vi "ABR3-Analyze.vi"(0 "Neural (uV)":dbl[](array[numeric]), 2 "Runtime":T1={"Ceiling"=0.0, "Threshold"=0.0, "Crossed?"=FALSE, "Step"=0, "Stop"=0, "Avgs"=0, "Level"=0.0, "AI Npts"=0, "Doubled?"=FALSE, "Gain"=0.0, "NWindowPts"=0, "dt"=0.0, "Cal"=path "", "Freq"=0.0, "AO Channels"=[], "AltPol"=FALSE, "AO Npts"=0, "AO Fs"=0.0, "Start"=0, "Stop max"=0, "Ear"=enum."Right", "Waveform"=enum."TONE PIP", "RepRate"=0.0, "CAP or ABR"=1, "LMasker"=0.0, "SeqVar"=enum."Signal Level", "Reps/buffer"=0, "Avg Mode"=enum."Neural/CM", "Wav"=path "", "Order"=enum."Sequential", "Levels"=[], "ControlVal"=0.0, "innerIndex"=0, "indexStep"=0} {"CAP or ABR" items=["CAP", "ABR"]}, 5 "microphonic (uV)":dbl[](array[numeric]), 7 "Averaging data":cluster{i32, i32}, 9 "Normalize individual?":bool, 11 "error in":errorcluster, 12 "Analysis":T6, 13 "Graphs":T5) -> (4 "spread value":dbl, 14 "Analysis out":T6, 15 "error out":errorcluster)   [LabVIEW 2020]
uses:
  TypeDefs/ABR3-Analysis State.ctl
  Threshold Estimation VIs/ABR3-Threshold Estimation Result.ctl
  TypeDefs/ABR3-Graph Controls.ctl
  TypeDefs/ABR3-Runtime Data.ctl
  epl-vi-lib/Utility VIs/Type Defs/Left-Right ring.ctl
  TypeDefs/ABR-Waveform Enum.ctl
  TypeDefs/ABR3-Seq Var Enum.ctl
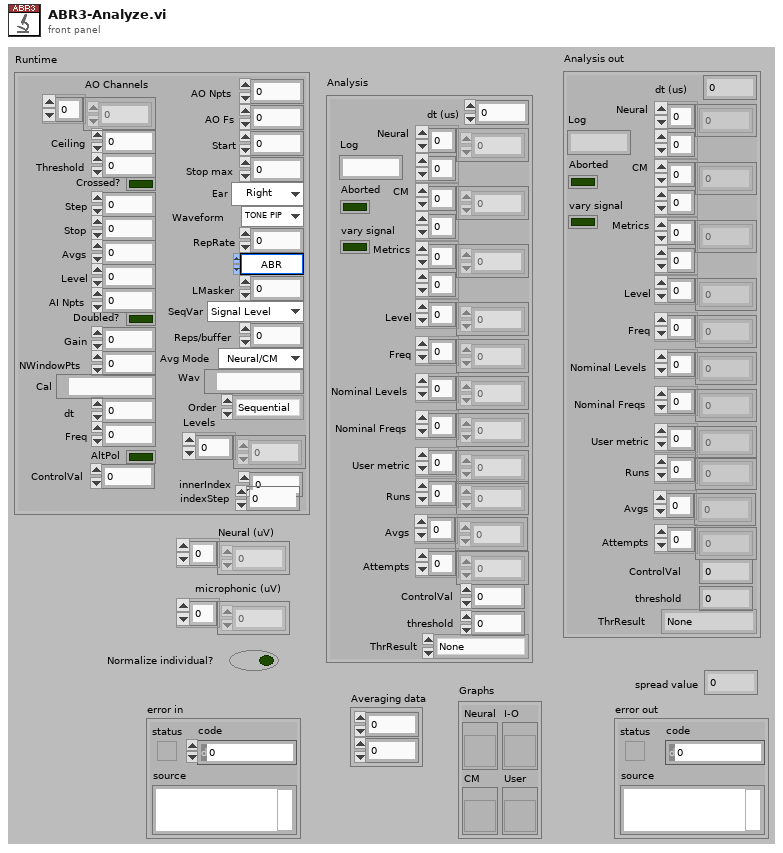
[diagram p1: front panel]
types:
  T1 = typedef "ABR3-Runtime Data.ctl" = cluster{"Ceiling":dbl, "Threshold":dbl, "Crossed?":bool, "Step":i32, "Stop":i32, "Avgs":i32, "Level":dbl, "AI Npts":i32, "Doubled?":bool, "Gain":dbl, "NWindowPts":i32, "dt":dbl, "Cal":path, "Freq":dbl, "AO Channels":i32[], "AltPol":bool, "AO Npts":i32, "AO Fs":dbl, "Start":i32, "Stop max":i32, "Ear":T2, "Waveform":T3, "RepRate":dbl, "CAP or ABR":u16, "LMasker":dbl, "SeqVar":T4, "Reps/buffer":i32, "Avg Mode":enum16{"Neural/CM", "ANOW"}, "Wav":path, "Order":enum16{"Sequential", "Random"}, "Levels":dbl[], "ControlVal":dbl, "innerIndex":i32, "indexStep":i32}
  T2 = typedef "Left-Right ring.ctl" = enum16{"Right", "Left"}
  T3 = typedef "ABR-Waveform Enum.ctl" = enum16{"TONE PIP", "CLICK", "FILE", "CHIRP", "NOISE", "VERHULST"}
  T4 = typedef "ABR3-Seq Var Enum.ctl" = enum16{"Signal Level", "Masker Level"}
  T5 = typedef "ABR3-Graph Controls.ctl" = cluster{"I-O":refnum<vi>, "Neural":refnum<vi>, "CM":refnum<vi>, "User":refnum<vi>}
  T6 = typedef "ABR3-Analysis State.ctl" = cluster{"dt (us)":dbl, "Neural":dbl[][], "CM":dbl[][], "Metrics":dbl[][], "Level":dbl[], "Freq":dbl[], "Nominal Levels":dbl[], "Nominal Freqs":dbl[], "User metric":dbl[], "Runs":i32[], "Avgs":i32[], "Attempts":i32[], "Log":string, "Aborted":bool, "ControlVal":dbl, "threshold":dbl, "vary signal":bool, "ThrResult":T7}
  T7 = typedef "ABR3-Threshold Estimation Result.ctl" = enum16{"None", "Power", "Sigmoid", "Power (noisy)", "Suprathreshold", "Invalid"}
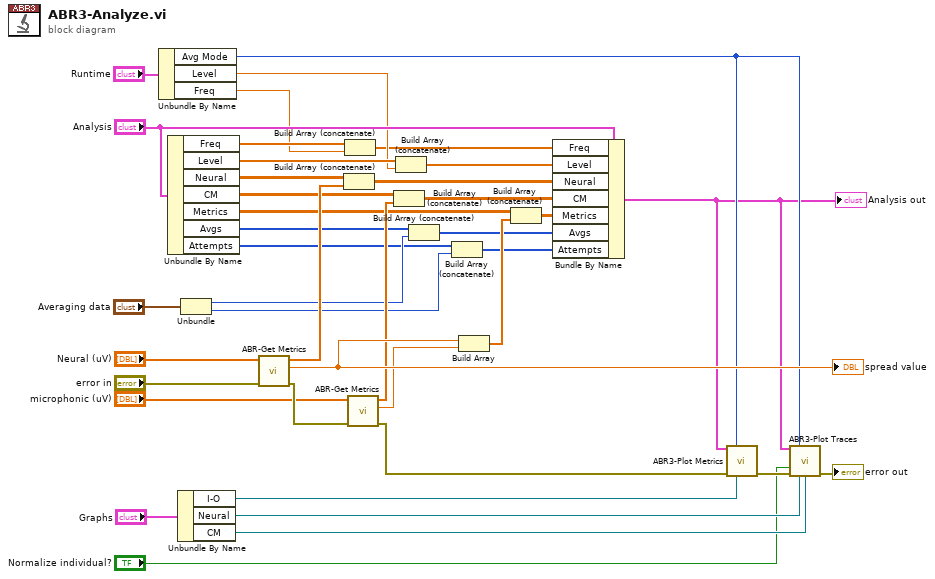
[diagram p0: block diagram]
diagram:
  n1 = Unbundle By Name("Runtime") -> ("Avg Mode"=w5:enum16{"Neural/CM", "ANOW"}, "Level"=w21:dbl, "Freq"=w24:dbl)
  n2 = Unbundle By Name("Analysis") -> ("Freq"=w25:dbl[], "Level"=w23:dbl[], "Neural"=w34:dbl[][], "CM"=w33:dbl[][], "Metrics"=w32:dbl[][], "Avgs"=w12:i32[], "Attempts"=w8:i32[])
  n3 = Unbundle By Name("Graphs") -> ("I-O"=w19:refnum<vi>, "Neural"=w16:refnum<vi>, "CM"=w15:refnum<vi>)
  n4 = Unbundle("Averaging data") -> (w10:i32, w6:i32)
  n5 = call "ABR-Get Metrics.vi"("error in (no error)"="error in", "Data in"="Neural (uV)") -> ("error out"=w27:errorcluster, "spread value"=w40:dbl, "Data out"=w38:dbl[])  [unwired: 7 in]
  "spread value" <- w40
  n6 = Build Array (concatenate)(w34, w38) -> (w30:dbl[][])
  n7 = Build Array (concatenate)(w25, w24) -> (w13:dbl[])
  n8 = call "ABR-Get Metrics.vi"("error in (no error)"=w27, "Data in"="microphonic (uV)") -> ("error out"=w4:errorcluster, "spread value"=w36:dbl, "Data out"=w37:dbl[])  [unwired: 7 in]
  n9 = Build Array (concatenate)(w33, w37) -> (w29:dbl[][])
  n10 = Build Array (concatenate)(w23, w21) -> (w22:dbl[])
  n11 = Build Array (concatenate)(w12, w10) -> (w9:i32[])
  n12 = Build Array (concatenate)(w8, w6) -> (w7:i32[])
  n13 = Build Array(w40, w36) -> (w39:dbl[])
  n14 = Build Array (concatenate)(w32, w39) -> (w28:dbl[][])
  n15 = Bundle By Name(cluster="Analysis", "Freq"=w13, "Level"=w22, "Neural"=w30, "CM"=w29, "Metrics"=w28, "Avgs"=w9, "Attempts"=w7) -> (w1:T6)
  "Analysis out" <- w1
  n16 = call "ABR3-Plot Metrics.vi"("Analysis"=w1, "Avg Mode"=w5, "error in (no error)"=w4, "I-O"=w19) -> ("error out"=w18:errorcluster)  [unwired: 11 in]
  n17 = call "ABR3-Plot Traces.vi"("Analysis"=w1, "Avg Mode"=w5, "Normalize individual?"="Normalize individual?", "error in (no error)"=w18, "Neural Ref"=w16, "CM Ref"=w15) -> ("error out"=→"error out":errorcluster)  [unwired: 9 in]
